vi "VISA shutter.vi"(8 "error in (no error)":errorcluster, 10 "button::shutter":bool, 11 "AOTF in":refnum<class "Invivo_AOTF.lvclass">) -> (0 "error out":errorcluster, 3 "AOTF out":refnum<class "Invivo_AOTF.lvclass">)   [LabVIEW 2012, in "Invivo_AOTF.lvclass"]
uses:
  Invivo_AOTF.lvclass
  Invivo_AOTF.lvclass/Invivo_AOTF.ctl
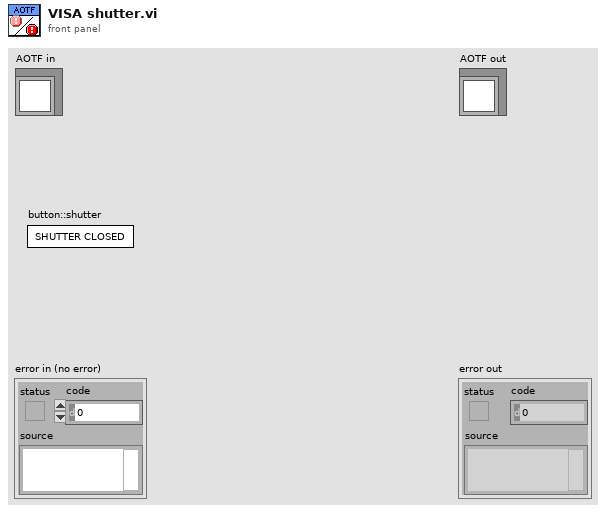
[diagram p1: front panel]
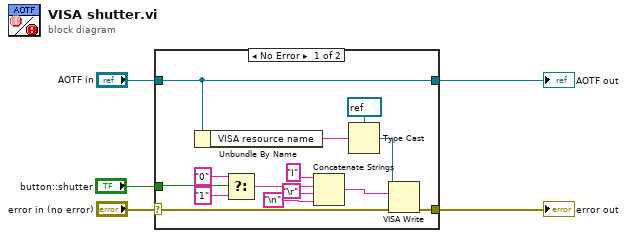
[diagram p0: block diagram]
diagram:
  n1 = case shown="No Error" "error in (no error)" {
    selector: "error in (no error)" -> [w9 w21]
    tunnel: [w8 w21] -> w4
    tunnel: [w19 w20] -> w2
    tunnel: "AOTF in" -> [w19 w20]
    tunnel: "button::shutter" -> [w13 _]
    frame No Error {
      n2 = Unbundle By Name(w19) -> ("VISA resource name"=w17:string)
      n3 = Select(t="0" ("string"), s=w13, f="1" ("string")) -> (s? t:f=w10:string)
      n4 = Concatenate Strings("I" ("string"), w10, "\r", "\n") -> (w7:string)
      n5 = Type Cast(type=refnum<visa-resource-name> refnum ("VISA resource name"), x=w17) -> (*(type *) &x=w14:refnum<visa-resource-name>)
      n6 = VISA Write(VISA resource name=w14, write buffer=w7, error in (no error)=w9) -> (error out=w8:errorcluster)  [unwired: 2 out]
    }
    frame Error {
    }
  }
  "error out" <- w4
  "AOTF out" <- w2
